vi "PulseTrain-Compute Max Level.vi"(0 "Pulse Train Params":T4, 5 "Filter":T3 {"IIR Filter Cluster"."Forward Coefficients" format="%.4f"; "IIR Filter Cluster"."Reverse Coefficients" format="%.4f"}, 9 "Level":T1, 11 "error in (no error)":errorcluster, 12 "Sampling Rate (Hz)":dbl, 13 "Npts":i32) -> (6 "Max Level":dbl, 10 "Level out":T1, 15 "error out":errorcluster)   [LabVIEW 2020]
uses:
  Pulse Train Params.ctl
  Pulse Polarity.ctl
  PT-Continuous State.ctl
  Controls/Filter XCtl/Filter Data.ctl
  Controls/Level XCtl/Level Data.ctl
  Controls/Level XCtl/Level Units.ctl
  <vilib>/Analysis/2dsp.llb/Inverse Complex FFT.vi
  PXI DAQ VIs/DAQ Engine VIs/PXI Globals.vi
  Utility VIs/Math VIs/Linear to dB (scalar).vi
  Utility VIs/Math VIs/dB to Linear (scalar).vi
  <vilib>/Analysis/NI_AALPro.lvlib
  Controls/Filter XCtl/Filter XCtl.xctl
  Controls/Level XCtl/Level XCtl.xctl
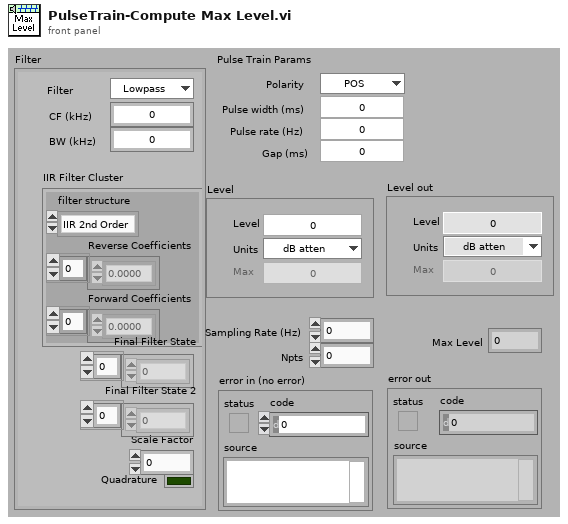
[diagram p1: front panel]
types:
  T1 = typedef "Level XCtl.xctl/Level Data.ctl" = cluster{"Level":dbl, "Units":T2, "Max":dbl, "Multiplier":dbl, "Cal File":path, "Cal":cluster{"Freq (Hz)":dbl[], "Mag (dB SPL)":dbl[], "Phase (deg)":dbl[]}}
  T2 = typedef "Level Units.ctl" = enum16{"dB atten", "dB SPL", "dB re 1 Vrms", "dB V/Hz½", "mW", "dB HL", "Volts", "dB mW"}
  T3 = typedef "Filter XCtl.xctl/Filter Data.ctl" = cluster{"CF (kHz)":dbl, "BW (kHz)":dbl, "IIR Filter Cluster":cluster{"filter structure":enum32{"IIR 2nd Order", "IIR 4th Order"}, "Reverse Coefficients":dbl[], "Forward Coefficients":dbl[]}, "Final Filter State":dbl[], "Scale Factor":dbl, "Final Filter State 2":dbl[], "Quadrature":bool, "Type":enum16{"Lowpass", "Highpass", "Bandpass", "Bandstop", "OFF"}}
  T4 = typedef "Pulse Train Params.ctl" = cluster{"Pulse width (us)":dbl, "Pulse rate (Hz)":dbl, "Gap (ms)":dbl, "Polarity":T5, "PT State":T6, "Asynch":bool}
  T5 = typedef "Pulse Polarity.ctl" = enum16{"POS", "NEG", "POS-NEG", "NEG-POS"}
  T6 = typedef "PT-Continuous State.ctl" = cluster{"Template":dbl[], "Nperiod":i32, "Index":i32, "Pulse Rate (Hz)":dbl, "Phase (cycles)":dbl, "Noff":i32}
  T7 = typedef "LaserCal-Data (I-O).ctl" = cluster{"I-O":cluster{dbl[], dbl[]}, "Time-Domain":cluster{dbl[], dbl[]}[], "Time Index":i32, "Data header":string, "Tsettle (s)":dbl}
  T8 = typedef "LaserCal-Data (PT).ctl" = cluster{"I-O":cluster{"Volts":dbl[], "Width":dbl[], "Rate":dbl[], "Power":dbl[][][][]}, "Data header":string, "Tsettle (s)":dbl}
  T9 = cluster{"Volts":dbl[], "Width":dbl[], "Rate":dbl[], "Power":dbl[][][][]}
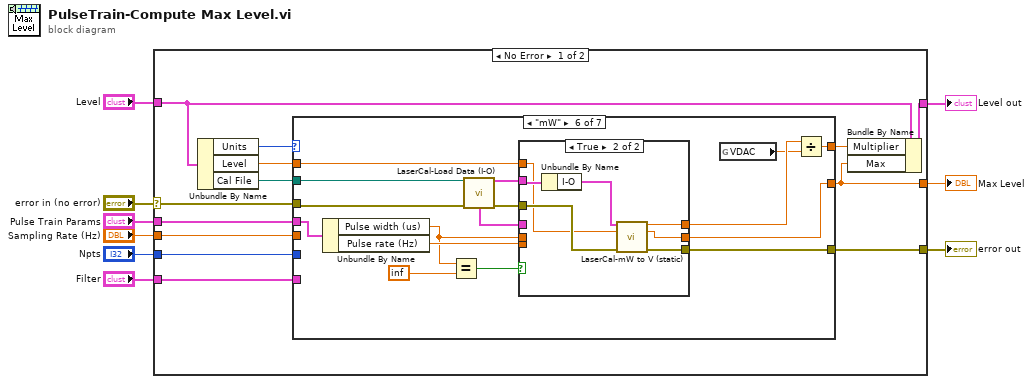
[diagram p0: block diagram]
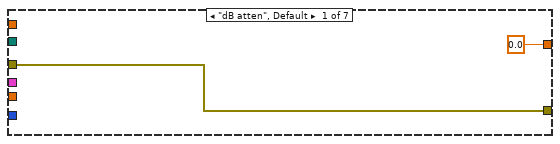
[diagram p2: hidden frame]
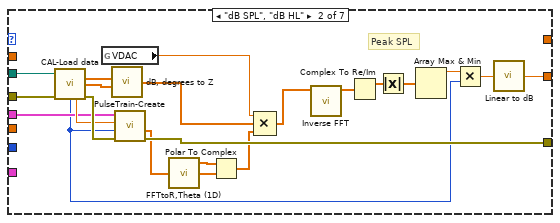
[diagram p3: hidden frame]
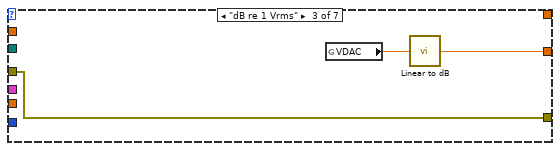
[diagram p4: hidden frame]
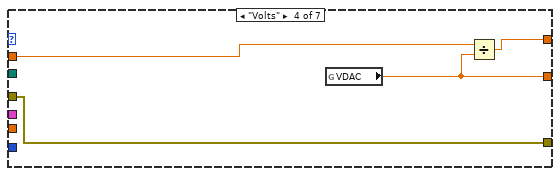
[diagram p5: hidden frame]
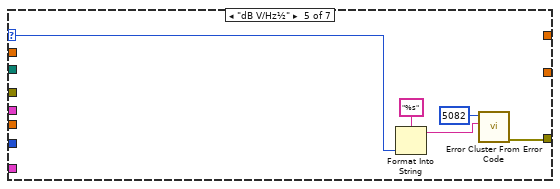
[diagram p6: hidden frame]
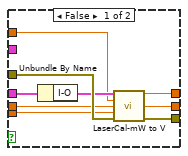
[diagram p7: hidden frame]
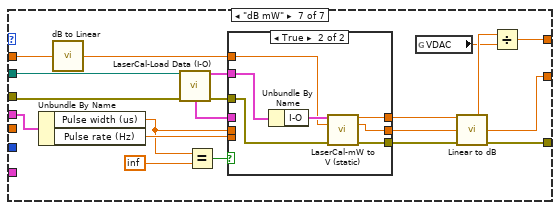
[diagram p8: hidden frame]
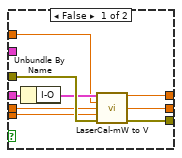
[diagram p9: hidden frame]
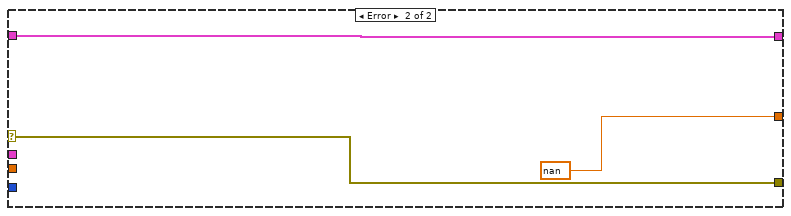
[diagram p10: hidden frame]
diagram:
  n1 = case shown="No Error" "error in (no error)" {
    selector: "error in (no error)" -> [w22 w127]
    tunnel: "Level" -> [w17 w125]
    tunnel: "Pulse Train Params" -> [w12 _]
    tunnel: "Filter" -> [w20 _]
    tunnel: [w18 w127] -> w8
    tunnel: "Npts" -> [w21 _]
    tunnel: [w16 nan ("Reference Level")] -> w3
    tunnel: "Sampling Rate (Hz)" -> [w19 _]
    tunnel: [w15 w125] -> w1
    frame No Error {
      n2 = Unbundle By Name(w17) -> ("Units"=w14:T2, "Level"=w10:dbl, "Cal File"=w13:path)
      n3 = case shown="\"mW\"" w14 {
        selector: w14 -> [_ _ _ _ w54 _ _]
        tunnel: w22 -> [w23 w46 w47 w53 _ w74 w108]
        tunnel: w21 -> [_ _ _ _ _ _ _]
        tunnel: w20 -> [_ _ _ _ _ _ _]
        tunnel: [0.0 ("Reference Level") w25 w48 w52 _ w68 w95] -> w16
        tunnel: w19 -> [_ _ _ _ _ _ _]
        tunnel: [w23 w39 w47 w53 w55 w71 w105] -> w18
        tunnel: w13 -> [_ w45 _ _ _ w64 w98]
        tunnel: w12 -> [_ w38 _ _ _ w73 w107]
        tunnel: [_ _ _ w50 _ w65 w99] -> w11
        tunnel: w10 -> [_ _ _ w51 _ w63 w97]
        frame "dB atten", Default {
        }
        frame "dB SPL", "dB HL" {
          # "Peak SPL"
          n4 = call "CAL-Load data.vi"("user path"=w45, "error in (no error)"=w46) -> ("Mag"=w44:dbl[], "Phase"=w43:dbl[], "npts"=w27:i32, "Fs (Hz)"=w40:dbl, "error out"=w41:errorcluster)  [unwired: 6 in, 3 out]
          n5 = global read "PXI Globals.vi" "VDAC"() -> (w37:dbl)
          n6 = call "dB, degrees to Z.vi"("Magnitude (dB)"=w44, "Phase (degrees)"=w43) -> ("Z"=w42:cdb[])  [unwired: 5 in]
          n7 = call "PulseTrain-Create.vi"("error in (no error)"=w41, "Npts"=w27, "Sampling Rate (Hz)"=w40, "Pulse Train Params"=w38) -> ("error out"=w39:errorcluster, "Waveform"=w36:dbl[])  [unwired: 4 in, 2 out]
          n8 = call "FFTtoR,Theta (1D).VI"("X"=w36) -> ("+Freq. Mag of FFT"=w34:dbl[], "+Freq Theta of FFT"=w35:dbl[])  [unwired: 1 in]
          n9 = Polar To Complex(1:w35, 2:w34) -> (0:w33:cdb[])
          n10 = Compound Arithmetic op=MULTIPLY(w37, w42, w33) -> (w32:cdb[])
          n11 = call-poly <vilib>:"Inverse FFT.vi"("FFT {X}"=w32) -> ("X"=w31:cdb[])  [unwired: 9 in, 1 out]
          n12 = Complex To Re/Im(x + iy=w31) -> (x=w30:dbl[])  [unwired: 1 out]
          n13 = Absolute Value(x=w30) -> (abs(x)=w28:dbl[])
          n14 = Array Max & Min(array=w28) -> (max value=w29:dbl)  [unwired: 3 out]
          n15 = Multiply(x=w29, y=w27) -> (x*y=w26:dbl)
          n16 = call-poly "Linear to dB.vi"("Linear"=w26) -> ("dB"=w25:dbl)
        }
        frame "dB re 1 Vrms" {
          n17 = global read "PXI Globals.vi" "VDAC"() -> (w49:dbl)
          n18 = call-poly "Linear to dB.vi"("Linear"=w49) -> ("dB"=w48:dbl)
        }
        frame "Volts" {
          n19 = global read "PXI Globals.vi" "VDAC"() -> (w52:dbl)
          n20 = Divide(x=w51, y=w52) -> (x/y=w50:dbl)
        }
        frame "dB V/Hz½" {
          n21 = Format Into String(format string="%s", w54) -> (resulting string=w57:string)  [unwired: 2 in, 1 out]
          n22 = call <vilib>:"Error Cluster From Error Code.vi"("error message (\"\")"=w57, "error code (0)"=5082) -> ("error out"=w55:errorcluster)  [unwired: 7 in]
        }
        frame "mW" {
          n23 = Unbundle By Name(w73) -> ("Pulse width (us)"=w60:dbl, "Pulse rate (Hz)"=w70:dbl)
          n24 = Equal?(x=w60, y=inf) -> (x = y?=w59:bool)
          n25 = call "LaserCal-Load Data (I-O).vi"("Path"=w64, "error in (no error)"=w74) -> ("I-O Data (static)"=w62:T7, "I-O Data"=w69:T8, "error out"=w72:errorcluster)  [unwired: 6 in, 5 out]
          n26 = case shown="True" w59 {
            tunnel: w72 -> [w83 w89]
            tunnel: [w82 w88] -> w71
            tunnel: w70 -> [w81 _]
            tunnel: w69 -> [w80 _]
            tunnel: w60 -> [w78 _]
            tunnel: [w77 w84] -> w68
            tunnel: [w76 w85] -> w67
            tunnel: w63 -> [w75 w86]
            tunnel: w62 -> [_ w90]
            frame False {
              n27 = Unbundle By Name(w80) -> ("I-O"=w79:T9)
              n28 = call "LaserCal-mW to V.vi"("I-O"=w79, "Power (mW)"=w75, "Pulse width (us)"=w78, "Pulse rate (Hz)"=w81, "error in (no error)"=w83) -> ("Volts"=w76:dbl, "Max (mW)"=w77:dbl, "error out"=w82:errorcluster)  [unwired: 8 in]
            }
            frame True {
              n29 = Unbundle By Name(w90) -> ("I-O"=w87:cluster{dbl[], dbl[]})
              n30 = call "LaserCal-mW to V (static).vi"("I-O"=w87, "Level"=w86, "error in (no error)"=w89) -> ("Voltage"=w85:dbl, "Max Power"=w84:dbl, "error out"=w88:errorcluster)  [unwired: 10 in]
            }
          }
          n31 = global read "PXI Globals.vi" "VDAC"() -> (w66:dbl)
          n32 = Divide(x=w67, y=w66) -> (x/y=w65:dbl)
        }
        frame "dB mW" {
          n33 = Unbundle By Name(w107) -> ("Pulse width (us)"=w94:dbl, "Pulse rate (Hz)"=w104:dbl)
          n34 = call-poly "dB to Linear.vi"("dB"=w97) -> ("linear"=w96:dbl)
          n35 = call "LaserCal-Load Data (I-O).vi"("Path"=w98, "error in (no error)"=w108) -> ("I-O Data (static)"=w92:T7, "I-O Data"=w103:T8, "error out"=w106:errorcluster)  [unwired: 6 in, 5 out]
          n36 = Equal?(x=w94, y=inf) -> (x = y?=w93:bool)
          n37 = case shown="True" w93 {
            tunnel: w106 -> [w117 w121]
            tunnel: [w116 w122] -> w105
            tunnel: w104 -> [w115 _]
            tunnel: w103 -> [w114 _]
            tunnel: w94 -> [w112 _]
            tunnel: [w111 w123] -> w102
            tunnel: [w110 w124] -> w101
            tunnel: w96 -> [w109 w118]
            tunnel: w92 -> [_ w120]
            frame False {
              n38 = Unbundle By Name(w114) -> ("I-O"=w113:T9)
              n39 = call "LaserCal-mW to V.vi"("I-O"=w113, "Power (mW)"=w109, "Pulse width (us)"=w112, "Pulse rate (Hz)"=w115, "error in (no error)"=w117) -> ("Volts"=w110:dbl, "Max (mW)"=w111:dbl, "error out"=w116:errorcluster)  [unwired: 8 in]
            }
            frame True {
              n40 = Unbundle By Name(w120) -> ("I-O"=w119:cluster{dbl[], dbl[]})
              n41 = call "LaserCal-mW to V (static).vi"("I-O"=w119, "Level"=w118, "error in (no error)"=w121) -> ("Voltage"=w124:dbl, "Max Power"=w123:dbl, "error out"=w122:errorcluster)  [unwired: 10 in]
            }
          }
          n42 = global read "PXI Globals.vi" "VDAC"() -> (w100:dbl)
          n43 = call-poly "Linear to dB.vi"("Linear"=w102) -> ("dB"=w95:dbl)
          n44 = Divide(x=w101, y=w100) -> (x/y=w99:dbl)
        }
      }
      n45 = Bundle By Name(cluster=w17, "Multiplier"=w11, "Max"=w16) -> (w15:T1)
    }
    frame Error {
    }
  }
  "error out" <- w8
  "Max Level" <- w3
  "Level out" <- w1
